vi "Test Include Dynamic Dispatch Method With Prefix.vi"(8 "error in (no error)":errorcluster, 11 "Test Case In":refnum<class "LUnit Test Suite Tests.lvclass">) -> (0 "error out":errorcluster, 3 "Test Case Out":refnum<class "LUnit Test Suite Tests.lvclass">)   [LabVIEW 2020, in "LUnit Test Suite Tests.lvclass"]
uses:
  LUnit Test Suite Tests.lvclass
  LUnit Test Suite Tests.lvclass/LUnit Test Suite Tests.ctl
  source/LUnit Test Suite.lvclass
  Test Doubles/Test Case Test Double/Test Case Test Double.lvclass
  82139866-69ca-4a01-bf4f-9813e5ee88f7.vi
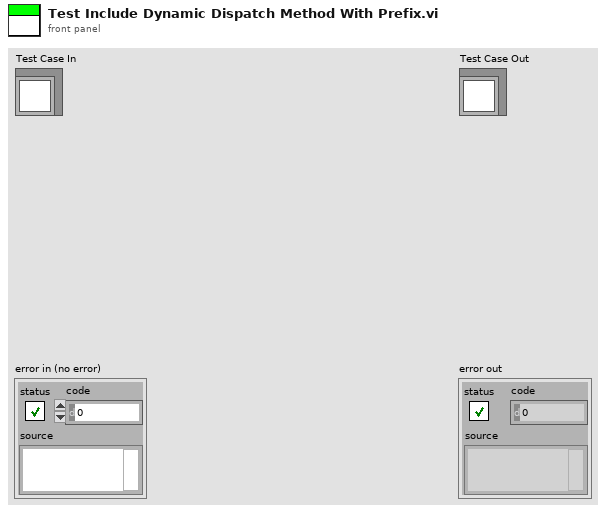
[diagram p1: front panel]
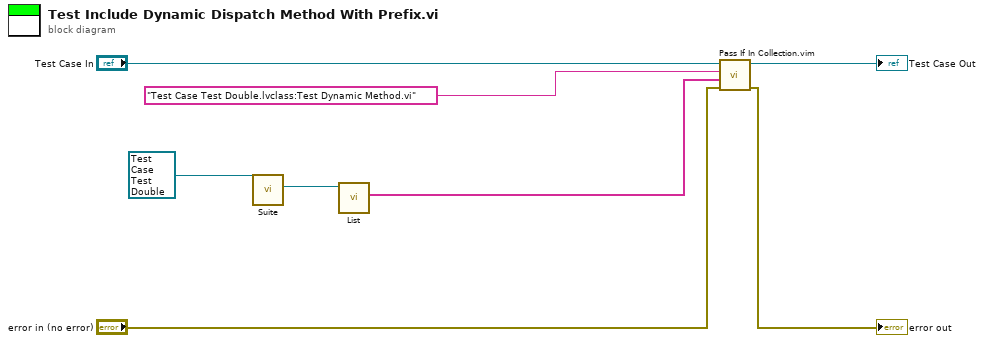
[diagram p0: block diagram]
diagram:
  n1 = call-dynamic "Suite.vi"("LUnit Test Case In"=refnum<class "Test Case Test Double.lvclass"> refnum ("Test Case Test Double.lvclass")) -> ("LUnit Test Suite Out"=w4:refnum<class "LUnit Test Suite.lvclass">)  [unwired: 8 in, 2 out]
  n2 = call "List.vi"("LUnit Test Suite In"=w4) -> ("List of Runnables"=w3:string[])  [unwired: 9 in, 1 out]
  n3 = call "Pass If In Collection.vim"("error in (no error)"="error in (no error)", "Collection"=w3, "Expected Element"="Test Case Test Double.lvclass:Test Dynamic Method.vi" ("String"), "LUnit Test Case In"="Test Case In") -> ("error out"=→"error out":errorcluster, "LUnit Test Case Out"=→"Test Case Out":refnum<class "LUnit Test Suite Tests.lvclass">)  [unwired: 6 in]
